vi "DIO Waveform Write.vi"(4 "Frequency":dbl=100000.0 caption="Frequency (Hz)" format="%0.2f", 6 "Counter":string, 8 "error in (no error)":errorcluster, 9 "Line":string, 10 "Port":string, 11 "DIO Device":tag) -> (0 "error out":errorcluster)   [LabVIEW 2022 SP3, in "niMIO.lvclass"]
uses:
  niMIO.lvclass
  <vilib>/DAQmx/write.llb/DAQmx Write (Digital Wfm 1Chan NSamp).vi
  <vilib>/Waveform/DWDTOps.llb/Digital Pattern Generator (Toggle).vi
  <vilib>/DAQmx/create/channels.llb/DAQmx Create Channel (CO-Pulse Generation-Frequency).vi
  <vilib>/DAQmx/configure/timing.llb/DAQmx Timing (Implicit).vi
  <vilib>/DAQmx/create/channels.llb/DAQmx Create Channel (DO-Digital Output).vi
  <vilib>/DAQmx/configure/timing.llb/DAQmx Timing (Sample Clock).vi
  <vilib>/Waveform/DWDTOps.llb/DWDT Uncompress Digital.vi
  <vilib>/DAQmx/miscellaneous.llb/DAQmx Fill In Error Info.vi
panel:
  out "niDIO out":refnum<class "niMIO.lvclass">
  in  "niDIO in":refnum<class "niMIO.lvclass">
  # "Digital Output Line"
  # "Timing Configuration"
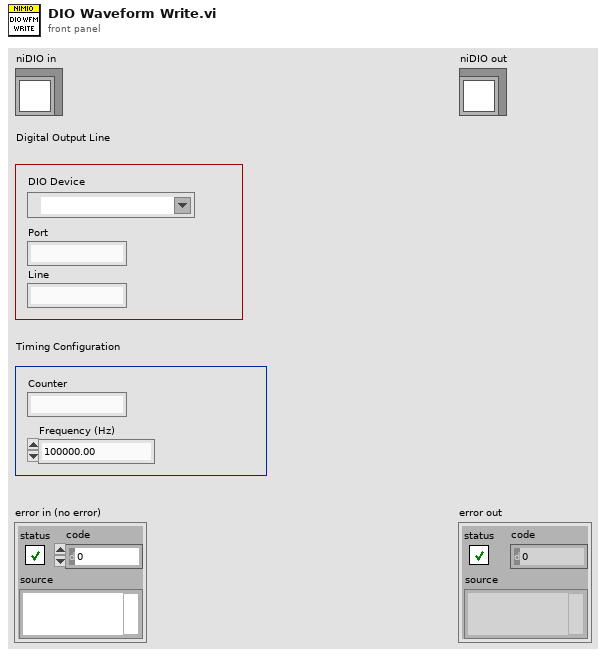
[diagram p1: front panel]
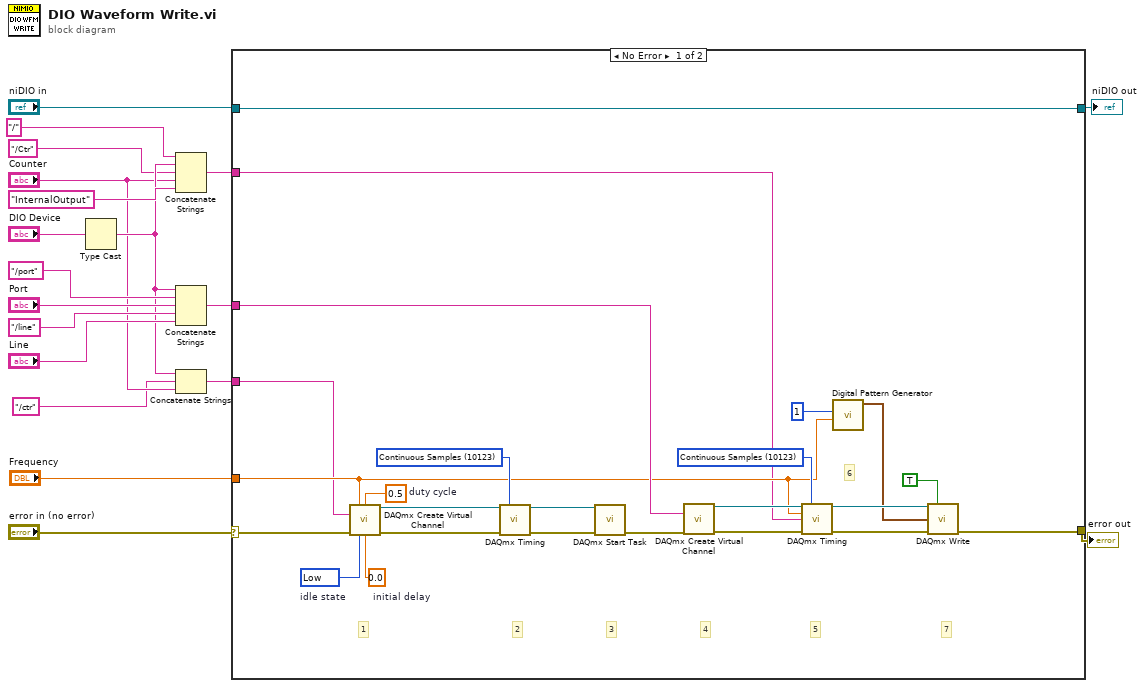
[diagram p0: block diagram]
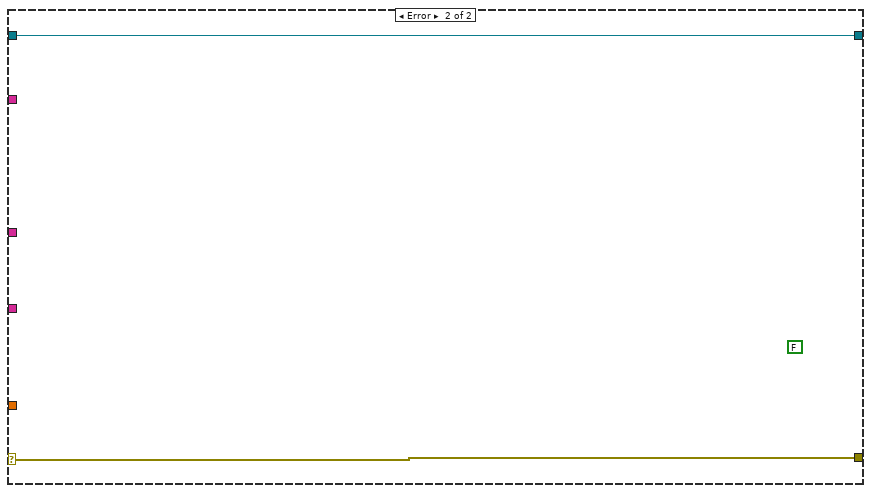
[diagram p2: hidden frame]
diagram:
  n1 = Type Cast(x="DIO Device") -> (*(type *) &x=w5:string)  [unwired: 1 in]
  n2 = Concatenate Strings("/" ("string"), w5, "/Ctr", "Counter", "InternalOutput") -> (w6:string)
  n3 = Concatenate Strings(w5, "/port", "Port", "/line" ("string"), "Line") -> (w11:string)
  n4 = Concatenate Strings(w5, "/ctr", "Counter") -> (w2:string)
  n5 = case shown="No Error" "error in (no error)" {
    selector: "error in (no error)" -> [w25 w45]
    tunnel: [w26 w45] -> w18
    tunnel: [w43 w44] -> w17
    tunnel: "niDIO in" -> [w43 w44]
    tunnel: w11 -> [w33 _]
    tunnel: "Frequency" -> [w23 _]
    tunnel: w6 -> [w21 _]
    tunnel: w2 -> [w20 _]
    frame No Error {
      w30 = 10123 items=["Finite Samples"=10178, "Continuous Samples"=10123, "Hardware Timed Single Point"=12522] ("sample mode")
      w37 = 10123 items=["Finite Samples"=10178, "Continuous Samples"=10123, "Hardware Timed Single Point"=12522] ("sample mode")
      w40 = 0.5  # duty cycle
      w41 = 0.0  # initial delay
      w42 = 10214 items=["High"=10192, "Low"=10214]  # idle state
      # "7"
      # "6"
      # "5"
      # "4"
      # "3"
      # "2"
      # "1"
      n6 = call-poly <vilib>:"DAQmx Create Virtual Channel.vi"("frequency"=w23, "duty cycle"=w40, "counter"=w20, "error in"=w25, "idle state"=w42, "initial delay"=w41) -> ("task out"=w38:refnum<k21>, "error out"=w39:errorcluster)  [unwired: 8 in]
      n7 = call-poly <vilib>:"DAQmx Timing.vi"("task/channels in"=w38, "sample mode"=w37, "error in"=w39) -> ("task out"=w36:refnum<k21>, "error out"=w35:errorcluster)  [unwired: 11 in]
      n8 = call <vilib>:"DAQmx Start Task.vi"("task/channels in"=w36, "error in"=w35) -> ("error out"=w34:errorcluster)  [unwired: 12 in, 1 out]
      n9 = call-poly <vilib>:"DAQmx Create Virtual Channel.vi"("lines"=w33, "error in"=w34) -> ("task out"=w32:refnum<k21>, "error out"=w31:errorcluster)  [unwired: 12 in]
      n10 = call-poly <vilib>:"DAQmx Timing.vi"("task/channels in"=w32, "sample mode"=w30, "rate"=w23, "source"=w21, "error in"=w31) -> ("task out"=w29:refnum<k21>, "error out"=w27:errorcluster)  [unwired: 9 in]
      n11 = call-poly <vilib>:"Digital Pattern Generator.vi"("sample rate"=w23, "number of signals"=u32 1) -> ("digital waveform"=w22:digitalwaveform)  [unwired: 8 in, 1 out]
      n12 = call-poly <vilib>:"DAQmx Write.vi"("task/channels in"=w29, "auto start"=TRUE, "data"=w22, "error in"=w27) -> ("error out"=w26:errorcluster)  [unwired: 9 in, 2 out]
    }
    frame Error {
      (unwired) FALSE ("data")
    }
  }
  "error out" <- w18
  "niDIO out" <- w17
